vi "Right manage.vi"() -> ()   [LabVIEW 2017]
uses:
  widgets/Popup/Popup.lvclass
panel:
  in  "Popup":T1 {"Right" items=["High", "Middle", "Low"]}
  in  "权限管理":i32(listbox)
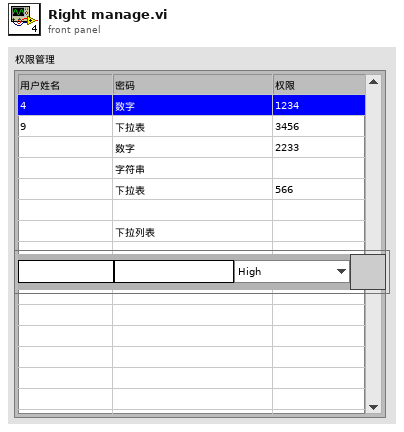
[diagram p1: front panel]
types:
  T1 = cluster{"Name":string, "Password":string, "Right":u16, "OK":bool}
  T2 = typedef "LVPoint32TypeDef.ctl" = cluster{"Horizontal":i32, "Vertical":i32}
  T3 = typedef "LVRowAndColumnTypeDef.ctl" = cluster{"Row":i32, "Column":i32}
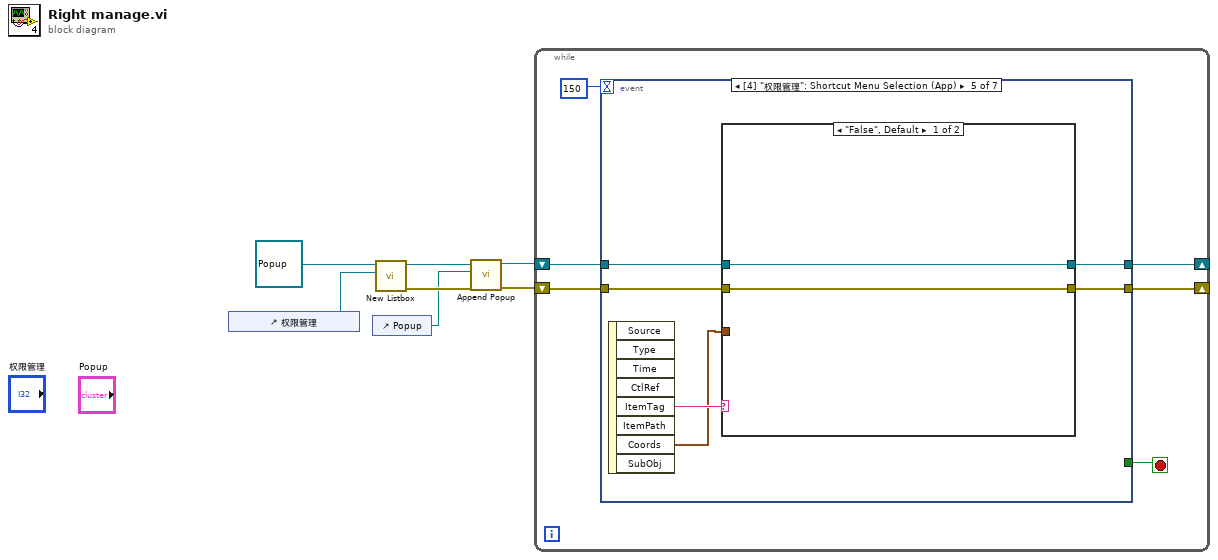
[diagram p0: block diagram]
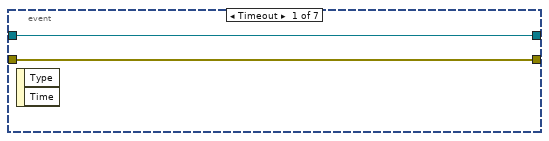
[diagram p2: hidden frame]
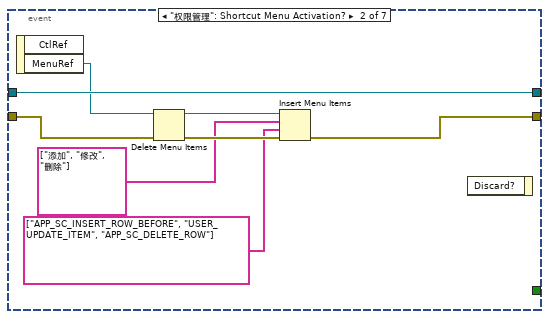
[diagram p3: hidden frame]
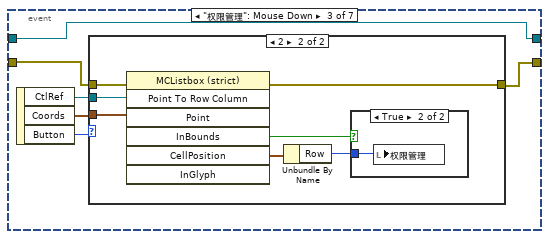
[diagram p4: hidden frame]
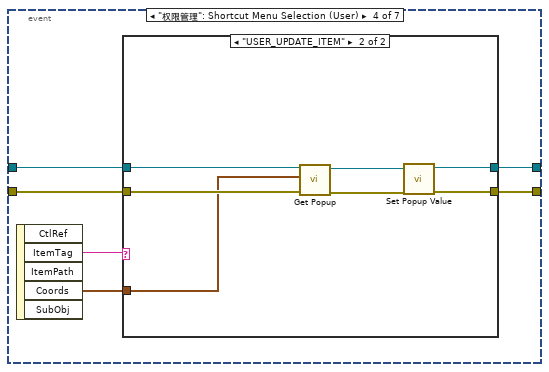
[diagram p7: hidden frame]
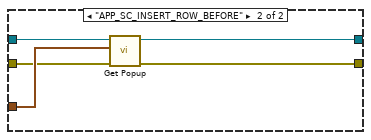
[diagram p9: hidden frame]
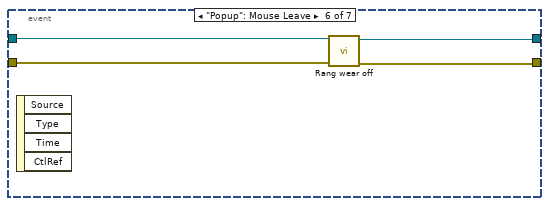
[diagram p10: hidden frame]
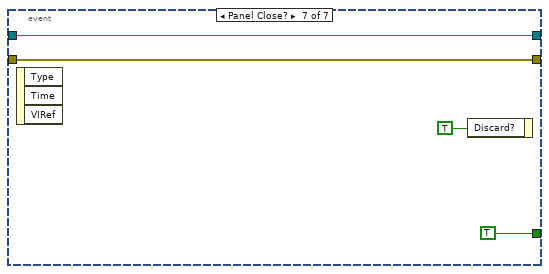
[diagram p11: hidden frame]
diagram:
  n1 = control-ref of="权限管理"() -> (w6:refnum<vi>)
  n2 = control-ref of="Popup"() -> (w3:refnum<vi>)
  n3 = call-dynamic "New Listbox.vi"("ListBox"=w6, "Popup 输入"=refnum<class "Popup.lvclass"> refnum) -> ("error out"=w4:errorcluster, "Popup 输出"=w5:refnum<class "Popup.lvclass">)  [unwired: 8 in]
  n4 = call-dynamic "Append Popup.vi"("error in (no error)"=w4, "PopupRef"=w3, "Popup 输入"=w5) -> ("error out"=w1:errorcluster, "Popup 输出"=w2:refnum<class "Popup.lvclass">)  [unwired: 7 in]
  n5 = while {
    shift-right: [w11] -> _
    shift-left: w1 -> [w13]
    shift-right: [w10] -> _
    shift-left: w2 -> [w9]
    stop <- w8 stop-if-true
    n6 = event shown="[4] \"权限管理\": Shortcut Menu Selection (App)" {
      selector: _ -> [_ _ _ _ _ _ _]
      dyn-events: _ -> [_ _ _ _ _ _ _]
      timeout: 150 -> [_ _ _ _ _ _ _]
      tunnel: w9 -> [w15 w22 w24 w43 w58 w70 w72]
      tunnel: w13 -> [w14 w21 w29 w42 w57 w69 w71]
      tunnel: [w14 w16 w27 w39 w54 w67 w71] -> w11
      tunnel: [w15 w22 w24 w40 w55 w68 w72] -> w10
      tunnel: [_ _ _ _ _ _ TRUE] -> w8
      event Timeout {
        n7 = event-data() -> ()  [unwired: 1 in, 2 out]
      }
      event "权限管理": Shortcut Menu Activation? {
        n8 = event-data() -> ("MenuRef"=w20:refnum<k9>)  [unwired: 1 in, 1 out]
        n9 = Delete Menu Items(6:w21, 9:w20) -> (0:w23:errorcluster, 3:w19:refnum<k9>)  [unwired: 2 in]
        n10 = Insert Menu Items(6:w23, 7:string[] ["APP_SC_INSERT_ROW_BEFORE", "USER_UPDATE_ITEM", "APP_SC_DELETE_ROW"], 8:string[] ["添加", "修改", "删除"], 9:w19) -> (0:w16:errorcluster)  [unwired: 2 in, 2 out]
        n11 = event-data() -> ()  [unwired: 2 in, 1 out]
      }
      event "权限管理": Mouse Down {
        n12 = event-data() -> ("CtlRef"=w28:refnum<vi>, "Coords"=w26:T2, "Button"=w25:u16)  [unwired: 1 in]
        n13 = case shown="2" w25 {
          tunnel: w26 -> [_ w34]
          tunnel: w28 -> [_ w37]
          tunnel: w29 -> [w30 w35]
          tunnel: [w30 w36] -> w27
          frame Default {
          }
          frame 2 {
            n14 = invoke class="MCListbox (strict)" method="Point To Row Column"(reference=w37, error in=w35, "Point"=w34) -> (error out=w36:errorcluster, "InBounds"=w33:bool, "CellPosition"=w32:T3)  [unwired: 4 in, 4 out]
            n15 = Unbundle By Name(w32) -> ("Row"=w31:i32)
            n16 = case shown="True" w33 {
              tunnel: w31 -> [_ w38]
              frame False {
              }
              frame True {
                n17 = local write "权限管理"(w38) -> ()
              }
            }
          }
        }
      }
      event "权限管理": Shortcut Menu Selection (User) {
        n18 = event-data() -> ("ItemTag"=w44:string, "Coords"=w41:T2)  [unwired: 1 in, 3 out]
        n19 = case shown="\"USER_UPDATE_ITEM\"" w44 {
          tunnel: w43 -> [w46 w53]
          tunnel: w42 -> [w45 w52]
          tunnel: w41 -> [_ w51]
          tunnel: [w46 w48] -> w40
          tunnel: [w45 w47] -> w39
          frame "False", Default {
          }
          frame "USER_UPDATE_ITEM" {
            n20 = call "Get Popup.vi"("error in (no error)"=w52, "Point"=w51, "Popup 输入"=w53) -> ("error out"=w49:errorcluster, "Popup 输出"=w50:refnum<class "Popup.lvclass">)  [unwired: 7 in]
            n21 = call-dynamic "Set Popup Value.vi"("error in (no error)"=w49, "Popup in"=w50) -> ("error out"=w47:errorcluster, "Popup out"=w48:refnum<class "Popup.lvclass">)  [unwired: 8 in]
          }
        }
      }
      event "权限管理": Shortcut Menu Selection (App) {
        n22 = event-data() -> ("ItemTag"=w59:string, "Coords"=w56:T2)  [unwired: 1 in, 6 out]
        n23 = case shown="\"False\", Default" w59 {
          tunnel: w58 -> [w61 w65]
          tunnel: w57 -> [w60 w64]
          tunnel: w56 -> [_ w66]
          tunnel: [w61 w63] -> w55
          tunnel: [w60 w62] -> w54
          frame "False", Default {
          }
          frame "APP_SC_INSERT_ROW_BEFORE" {
            n24 = call "Get Popup.vi"("error in (no error)"=w64, "Point"=w66, "Popup 输入"=w65) -> ("error out"=w62:errorcluster, "Popup 输出"=w63:refnum<class "Popup.lvclass">)  [unwired: 7 in]
          }
        }
      }
      event "Popup": Mouse Leave {
        n25 = event-data() -> ()  [unwired: 1 in, 4 out]
        n26 = call-dynamic "Rang wear off.vi"("error in (no error)"=w69, "Popup 输入"=w70) -> ("error out"=w67:errorcluster, "Popup 输出"=w68:refnum<class "Popup.lvclass">)  [unwired: 8 in]
      }
      event Panel Close? {
        n27 = event-data() -> ()  [unwired: 1 in, 3 out]
        n28 = event-data("Discard?"=TRUE) -> ()  [unwired: 1 in, 1 out]
      }
    }
  }
